vi "CompareElements.vi"(8 "right":string, 11 "left":string) -> (1 "not equal":bool, 3 "in order":bool)   [LabVIEW 2023]
panel:
  out "pop right":string
  out "pop left":string
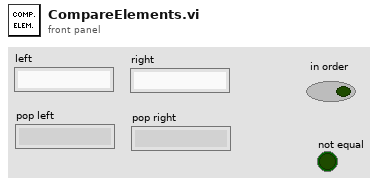
[diagram p1: front panel]
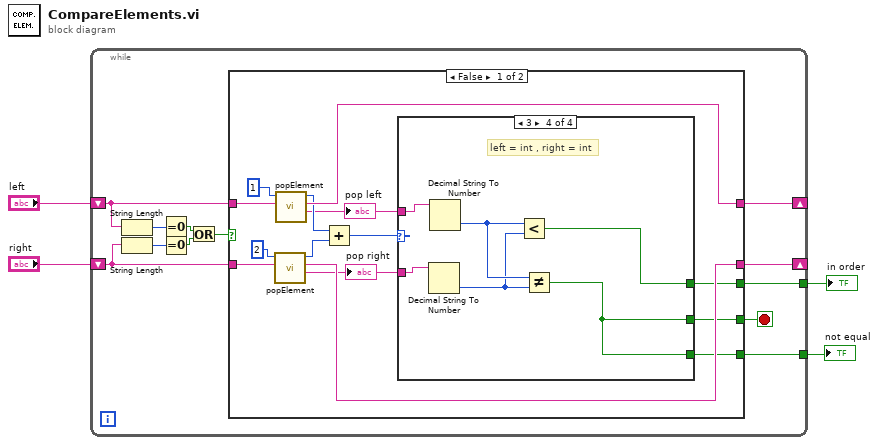
[diagram p0: block diagram]
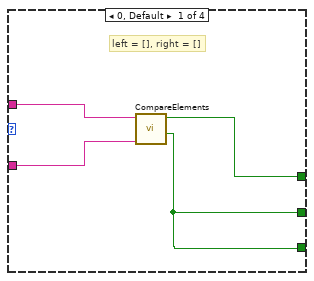
[diagram p2: hidden frame]
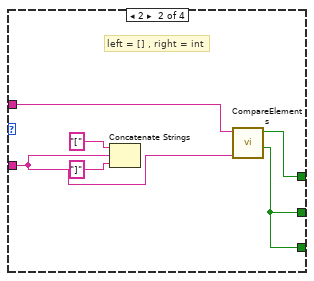
[diagram p3: hidden frame]
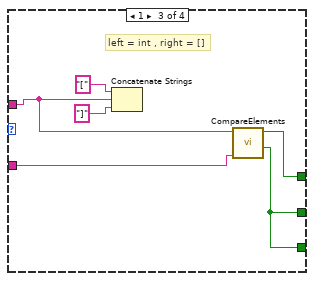
[diagram p4: hidden frame]
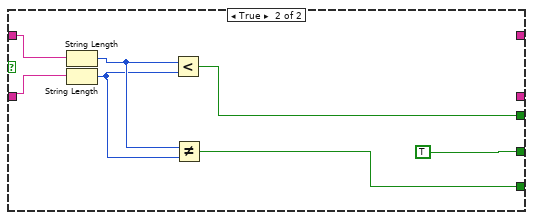
[diagram p5: hidden frame]
diagram:
  n1 = while {
    shift-right: [w16] -> _
    shift-left: "left" -> [w13]
    shift-right: [w15] -> _
    shift-left: "right" -> [w12]
    tunnel: [w14] -> w4
    tunnel: [w5] -> w1
    stop <- w6 stop-if-true
    n2 = String Length(string=w13) -> (length=w11:i32)
    n3 = String Length(string=w12) -> (length=w10:i32)
    n4 = Equal To 0?(x=w11) -> (x = 0?=w8:bool)
    n5 = Equal To 0?(x=w10) -> (x = 0?=w9:bool)
    n6 = Or(x=w8, y=w9) -> (x .or. y?=w7:bool)
    n7 = case shown="False" w7 {
      tunnel: [w29 _] -> w16
      tunnel: [w27 _] -> w15
      tunnel: [w23 TRUE] -> w6
      tunnel: [w22 w57] -> w14
      tunnel: w13 -> [w21 w59]
      tunnel: w12 -> [w20 w58]
      tunnel: [w19 w54] -> w5
      frame False {
        n8 = call "popElement.vi"("result string 3"=w20, "type in"=2 ("type")) -> ("element"=w17:string, "rest"=w27:string, "type out"=w25:i32)  [unwired: 7 in]
        "pop right" <- w17
        n9 = call "popElement.vi"("result string 3"=w21, "type in"=1 ("type")) -> ("element"=w18:string, "rest"=w29:string, "type out"=w26:i32)  [unwired: 7 in]
        "pop left" <- w18
        n10 = Add(x=w26, y=w25) -> (x+y=w24:i32)
        n11 = case shown="3" w24 {
          tunnel: w18 -> [w34 w40 w41 w52]
          tunnel: w17 -> [w33 w35 w42 w51]
          tunnel: [w31 w38 w45 w47] -> w23
          tunnel: [w32 w39 w46 w48] -> w22
          tunnel: [w31 w38 w45 w47] -> w19
          frame 0, Default {
            # "left = [], right = []"
            n12 = call "CompareElements.vi"("right"=w33, "left"=w34) -> ("not equal"=w31:bool, "in order"=w32:bool)  [unwired: 8 in]
          }
          frame 2 {
            # "left = [] , right = int"
            n13 = Concatenate Strings("[" ("string"), w35, "]" ("string")) -> ()  [unwired: 1 out]
            n14 = call "CompareElements.vi"("right"=w35, "left"=w40) -> ("not equal"=w38:bool, "in order"=w39:bool)  [unwired: 8 in]
          }
          frame 1 {
            # "left = int , right = []"
            n15 = Concatenate Strings("[" ("string"), w41, "]" ("string")) -> ()  [unwired: 1 out]
            n16 = call "CompareElements.vi"("right"=w42, "left"=w41) -> ("not equal"=w45:bool, "in order"=w46:bool)  [unwired: 8 in]
          }
          frame 3 {
            # "left = int , right = int"
            n17 = Decimal String To Number(string=w51) -> (number=w49:i32)  [unwired: 2 in, 1 out]
            n18 = Decimal String To Number(string=w52) -> (number=w50:i32)  [unwired: 2 in, 1 out]
            n19 = Less?(x=w50, y=w49) -> (x < y?=w48:bool)
            n20 = Not Equal?(x=w50, y=w49) -> (x != y?=w47:bool)
          }
        }
      }
      frame True {
        n21 = String Length(string=w59) -> (length=w56:i32)
        n22 = String Length(string=w58) -> (length=w55:i32)
        n23 = Less?(x=w56, y=w55) -> (x < y?=w57:bool)
        n24 = Not Equal?(x=w56, y=w55) -> (x != y?=w54:bool)
      }
    }
  }
  "in order" <- w4
  "not equal" <- w1
